vi "Pic Crop.vi"(8 "error in (no error)":errorcluster, 10 "Position":T1, 11 "24-bit pixmap in":u32[][](array[numeric]) format="%x") -> (0 "error out":errorcluster, 3 "24-bit pixmap out":u32[][](array[numeric]) format="%x")   [LabVIEW 2018, in "Picture Process.lvclass"]
uses:
  Picture Process.lvclass
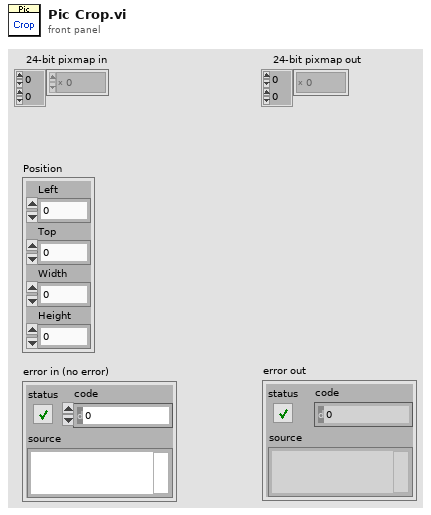
[diagram p1: front panel]
types:
  T1 = cluster{"Left":i16, "Top":i16, "Width":i16, "Height":i16}
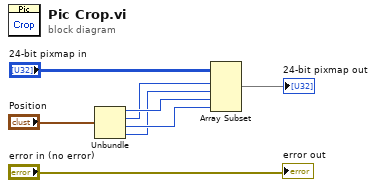
[diagram p0: block diagram]
diagram:
  n1 = Unbundle("Position") -> ("Left"=w4:i16, "Top"=w2:i16, "Width"=w3:i16, "Height"=w1:i16)
  n2 = Array Subset(array="24-bit pixmap in", index (row)=w2, length (row)=w1, index (col)=w4, length (col)=w3) -> (→"24-bit pixmap out":u32[][])
  "error out" <- "error in (no error)"
